vi "RH Calculate.vi"(10 "T_饱和":sgl, 11 "T_露点":sgl) -> (1 "Pws":sgl, 2 "Pw":sgl, 3 "RH(%)":sgl)   [LabVIEW 2020]
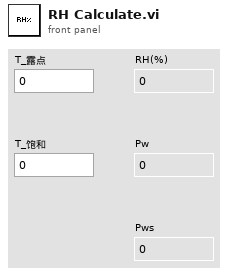
[diagram p1: front panel]
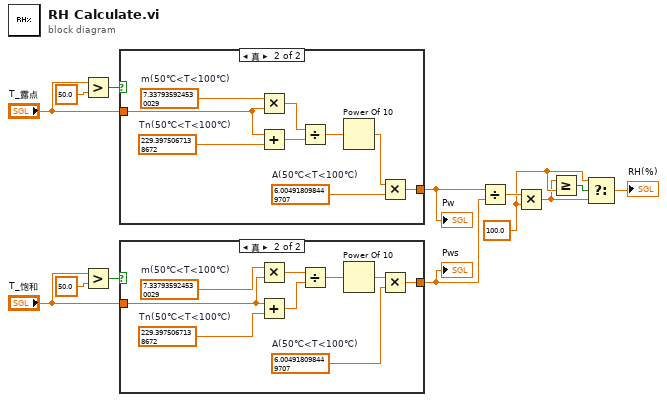
[diagram p0: block diagram]
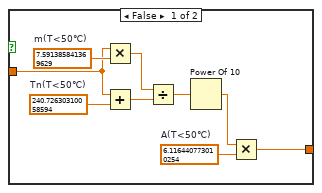
[diagram p2: hidden frame]
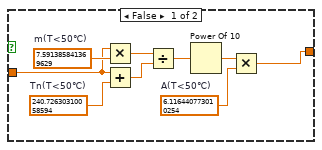
[diagram p3: hidden frame]
diagram:
  w3 = sgl 100.0 ("y")
  n1 = Greater?(x="T_露点", y=sgl 50.0) -> (0:w10:bool)
  n2 = Greater?(x="T_饱和", y=sgl 50.0) -> (0:w6:bool)
  n3 = case shown="真" w10 {
    tunnel: "T_露点" -> [w17 w29]
    tunnel: [w14 w23] -> w8
    frame False {
      w15 = sgl 6.116441  # A(T<50℃)
      w16 = sgl 240.7263  # Tn(T<50℃)
      w18 = sgl 7.591386  # m(T<50℃)
      n4 = Multiply(x=w17, y=w18) -> (x*y=w22:sgl)
      n5 = Add(x=w17, y=w16) -> (x+y=w21:sgl)
      n6 = Divide(x=w22, y=w21) -> (x/y=w20:sgl)
      n7 = Power Of 10(x=w20) -> (10^x=w19:sgl)
      n8 = Multiply(x=w19, y=w15) -> (x*y=w14:sgl)
    }
    frame True {
      w28 = sgl 229.3975  # Tn(50℃<T<100℃)
      w31 = sgl 7.337936  # m(50℃<T<100℃)
      w24 = sgl 6.004918  # A(50℃<T<100℃)
      n9 = Multiply(x=w31, y=w29) -> (x*y=w30:sgl)
      n10 = Add(x=w29, y=w28) -> (x+y=w27:sgl)
      n11 = Divide(x=w30, y=w27) -> (x/y=w26:sgl)
      n12 = Power Of 10(x=w26) -> (10^x=w25:sgl)
      n13 = Multiply(x=w25, y=w24) -> (x*y=w23:sgl)
    }
  }
  "Pw" <- w8
  n14 = case shown="真" w6 {
    tunnel: [w33 w42] -> w5
    tunnel: "T_饱和" -> [w32 w41]
    frame False {
      w34 = sgl 6.116441  # A(T<50℃)
      w35 = sgl 240.7263  # Tn(T<50℃)
      w36 = sgl 7.591386  # m(T<50℃)
      n15 = Multiply(x=w32, y=w36) -> (x*y=w40:sgl)
      n16 = Add(x=w32, y=w35) -> (x+y=w39:sgl)
      n17 = Divide(x=w40, y=w39) -> (x/y=w38:sgl)
      n18 = Power Of 10(x=w38) -> (10^x=w37:sgl)
      n19 = Multiply(x=w37, y=w34) -> (x*y=w33:sgl)
    }
    frame True {
      w47 = sgl 229.3975  # Tn(50℃<T<100℃)
      w49 = sgl 7.337936  # m(50℃<T<100℃)
      w43 = sgl 6.004918  # A(50℃<T<100℃)
      n20 = Multiply(x=w49, y=w41) -> (x*y=w48:sgl)
      n21 = Add(x=w41, y=w47) -> (x+y=w46:sgl)
      n22 = Divide(x=w48, y=w46) -> (x/y=w45:sgl)
      n23 = Power Of 10(x=w45) -> (10^x=w44:sgl)
      n24 = Multiply(x=w44, y=w43) -> (x*y=w42:sgl)
    }
  }
  "Pws" <- w5
  n25 = Divide(x=w8, y=w5) -> (x/y=w7:sgl)
  n26 = Multiply(x=w7, y=w3) -> (x*y=w2:sgl)
  n27 = Greater Or Equal?(x=w2, y=w3) -> (x >= y?=w4:bool)
  n28 = Select(t=w3, s=w4, f=w2) -> (s? t:f=→"RH(%)":sgl)
